vi "NtfyLvFpga_SUB_ValidationSmtpConfig.vi"(10 "Config":T1={"SMTP Setting"={"smtp server"="", "From"="", "port number"=25, "chk smtp auth"=FALSE, "userID"="", "password"="", "chk ssl"=FALSE}, "SendTo"={"To 1"={"chk"=FALSE, "To"=""}, "To 2"={"chk"=FALSE, "To"=""}, "To 3"={"chk"=FALSE, "To"=""}}, "Prohibit time"={"chk enable"=FALSE, "start hour"=0, "end hour"=0}}) -> (2 "Valid?":bool)   [LabVIEW 2013]
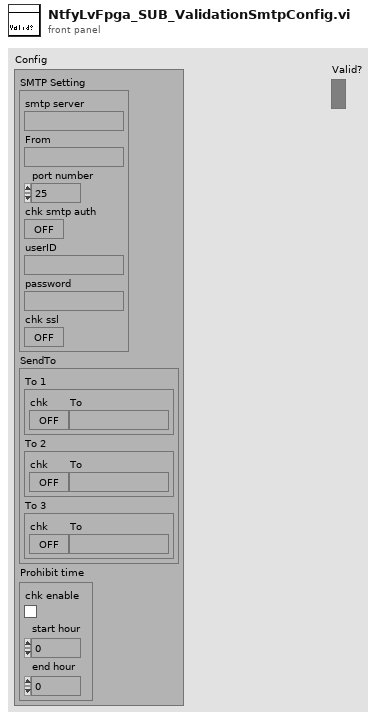
[diagram p1: front panel]
types:
  T1 = cluster{"SMTP Setting":cluster{"smtp server":string, "From":string, "port number":i32, "chk smtp auth":bool, "userID":string, "password":string, "chk ssl":bool}, "SendTo":cluster{"To 1":cluster{"chk":bool, "To":string}, "To 2":cluster{"chk":bool, "To":string}, "To 3":cluster{"chk":bool, "To":string}}, "Prohibit time":cluster{"chk enable":bool, "start hour":u8, "end hour":u8}}
  T2 = cluster{"smtp server":string, "From":string, "port number":i32, "chk smtp auth":bool, "userID":string, "password":string, "chk ssl":bool}
  T3 = cluster{"To 1":cluster{"chk":bool, "To":string}, "To 2":cluster{"chk":bool, "To":string}, "To 3":cluster{"chk":bool, "To":string}}
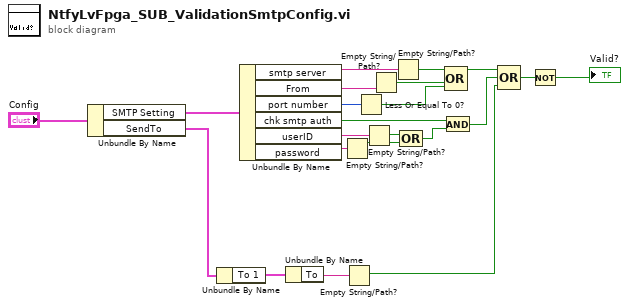
[diagram p0: block diagram]
diagram:
  n1 = Unbundle By Name("Config") -> ("SMTP Setting"=w21:T2, "SendTo"=w20:T3)
  n2 = Unbundle By Name(w20) -> ("To 1"=w19:cluster{"chk":bool, "To":string})
  n3 = Unbundle By Name(w21) -> ("smtp server"=w17:string, "From"=w16:string, "port number"=w18:i32, "chk smtp auth"=w12:bool, "userID"=w11:string, "password"=w10:string)
  n4 = Unbundle By Name(w19) -> ("To"=w4:string)
  n5 = Empty String/Path?(string/path=w10) -> (empty?=w8:bool)
  n6 = Empty String/Path?(string/path=w4) -> (empty?=w3:bool)
  n7 = Less Or Equal To 0?(x=w18) -> (x <= 0?=w13:bool)
  n8 = Empty String/Path?(string/path=w11) -> (empty?=w9:bool)
  n9 = Empty String/Path?(string/path=w16) -> (empty?=w14:bool)
  n10 = Empty String/Path?(string/path=w17) -> (empty?=w15:bool)
  n11 = Compound Arithmetic op=OR(w9, w8) -> (w7:bool)
  n12 = And(x=w12, y=w7) -> (x .and. y?=w5:bool)
  n13 = Compound Arithmetic op=OR(w15, w14, w13) -> (w6:bool)
  n14 = Compound Arithmetic op=OR(w6, w5, w3) -> (w2:bool)
  n15 = Not(x=w2) -> (.not. x?=→"Valid?":bool)
